vi "Create UTF-8 String.vi"(8 "error in (no error)":errorcluster, 11 "UTF-8 String":string) -> (0 "error out":errorcluster, 3 "UTF-8 String":refnum<class "UTF-8 String.lvclass">)   [LabVIEW 2010, in "JKI Unicode.lvlib" / "UTF-8 String.lvclass"]
uses:
  UTF-8 String.lvclass
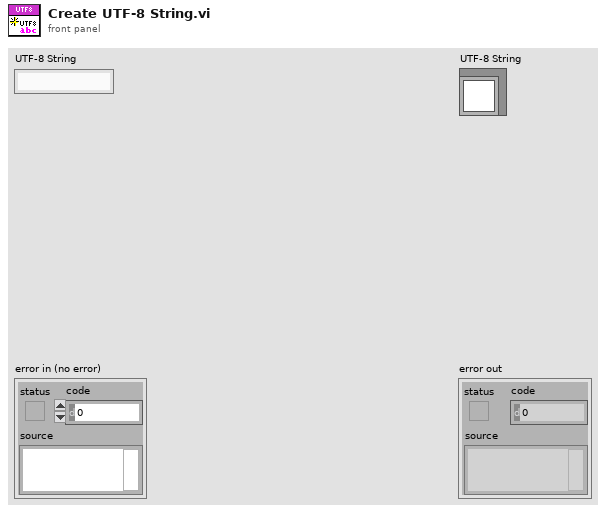
[diagram p1: front panel]
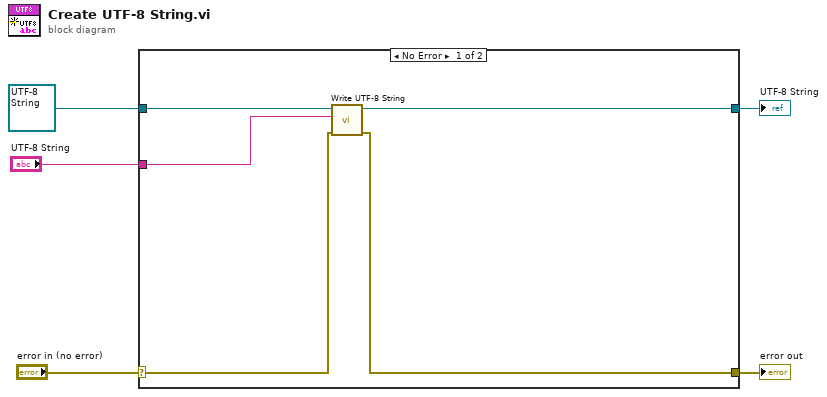
[diagram p0: block diagram]
diagram:
  n1 = case shown="No Error" "error in (no error)" {
    selector: "error in (no error)" -> [w8 w12]
    tunnel: [w7 w12] -> w4
    tunnel: [w9 w11] -> w2
    tunnel: refnum<class "UTF-8 String.lvclass"> refnum ("UTF-8 String in") -> [w10 w11]
    tunnel: "UTF-8 String" -> [w6 _]
    frame No Error {
      n2 = call-dynamic "Write UTF-8 String.vi"("error in (no error)"=w8, "UTF-8 String"=w6, "UTF-8 String in"=w10) -> ("error out"=w7:errorcluster, "UTF-8 String out"=w9:refnum<class "UTF-8 String.lvclass">)  [unwired: 7 in]
    }
    frame Error {
    }
  }
  "error out" <- w4
  "UTF-8 String" <- w2
